vi "Close File.vi"(8 "error in":errorcluster, 11 "TDMS in":refnum<class "TDMS.lvclass">) -> (0 "error out":errorcluster, 3 "TDMS out":refnum<class "TDMS.lvclass">)   [LabVIEW 2017, in "Report_lib.lvlib" / "TDMS.lvclass"]
uses:
  TDMS.lvclass
  TDMS.lvclass/TDMS.ctl
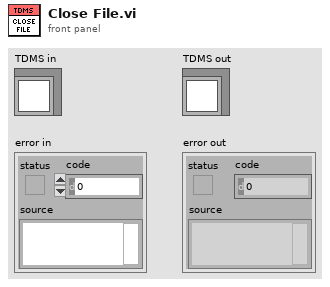
[diagram p1: front panel]
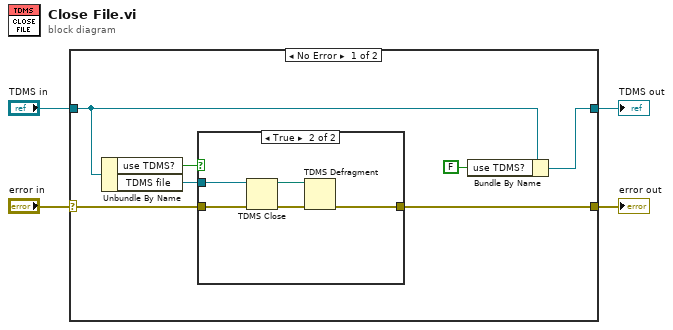
[diagram p0: block diagram]
diagram:
  n1 = case shown="No Error" "error in" {
    selector: "error in" -> [w9 w19]
    tunnel: [w8 w19] -> w3
    tunnel: [w5 w18] -> w1
    tunnel: "TDMS in" -> [w6 w18]
    frame No Error {
      n2 = Unbundle By Name(w6) -> ("use TDMS?"=w11:bool, "TDMS file"=w10:refnum<k34>)
      n3 = case shown="True" w11 {
        tunnel: w10 -> [_ w15]
        tunnel: w9 -> [w12 w14]
        tunnel: [w12 w13] -> w8
        frame False {
        }
        frame True {
          n4 = TDMS Close(8:w14, 11:w15) -> (0:w17:errorcluster, 3:w16:path)
          n5 = TDMS Defragment(4:w17, 7:w16) -> (0:w13:errorcluster)
        }
      }
      n6 = Bundle By Name(cluster=w6, "use TDMS?"=FALSE) -> (w5:refnum<class "TDMS.lvclass">)
    }
    frame Error {
    }
  }
  "error out" <- w3
  "TDMS out" <- w1
